vi "Data.vi"(7 "Data Type":T1(ring), 8 "Error In":errorcluster, 11 "Read Buffer":string) -> (0 "Error Out":errorcluster, 3 "XYZ":T2)   [LabVIEW 2010]
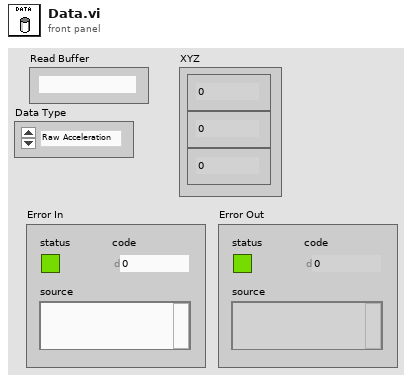
[diagram p1: front panel]
types:
  T1 = enum16{"Raw Acceleration", "Raw Gyro", "Complementy Filter", "Kalman Filter"}
  T2 = cluster{"Numeric Control":dbl, "Numeric Control":dbl, "Numeric Control":dbl}
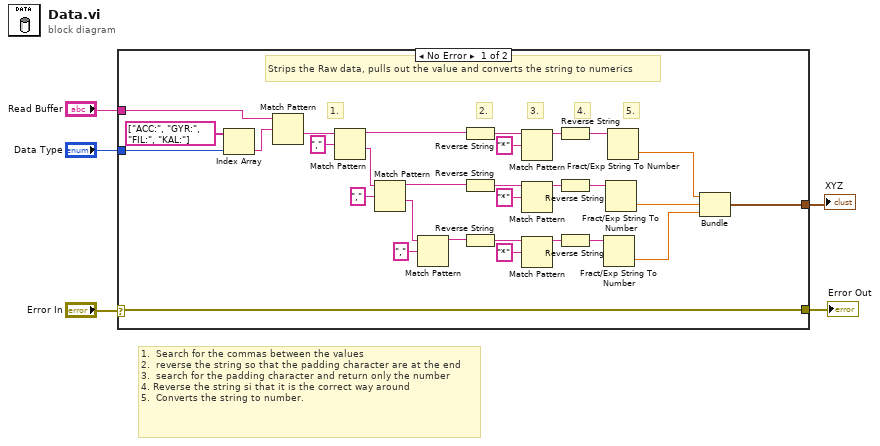
[diagram p0: block diagram]
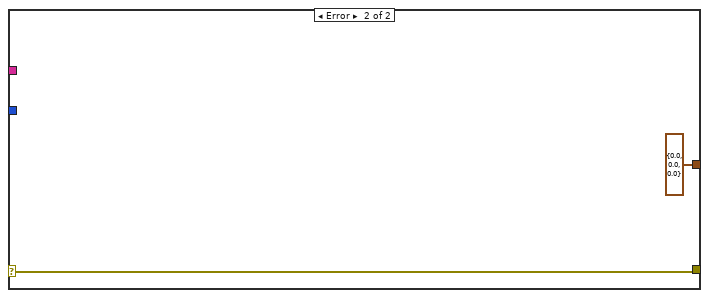
[diagram p2: hidden frame]
diagram:
  # "1.  Search for the commas between the values\n2.  reverse the string so that the padding character are at the end\n3.  search for the padding character and return only the number\n4. Reverse the string si that it is the correct way around\n5.  Converts the string to number."
  n1 = case shown="No Error" "Error In" {
    selector: "Error In" -> [w11 w37]
    tunnel: [w11 w37] -> w4
    tunnel: "Read Buffer" -> [w10 _]
    tunnel: [w9 cluster{dbl, dbl, dbl} {0.0, 0.0, 0.0}] -> w2
    tunnel: "Data Type" -> [w7 _]
    frame No Error {
      # "5."
      # "4."
      # "3."
      # "2."
      # "1."
      # "Strips the Raw data, pulls out the value and converts the string to numerics"
      n2 = Index Array(array=string[] ["ACC:", "GYR:", "FIL:", "KAL:"], index=w7) -> (element=w6:string)
      n3 = Match Pattern(string=w10, regular expression=w6) -> (after substring=w12:string)  [unwired: 1 in, 3 out]
      n4 = Match Pattern(string=w12, regular expression=",") -> (before substring=w14:string, after substring=w23:string)  [unwired: 1 in, 2 out]
      n5 = Match Pattern(string=w23, regular expression=",") -> (before substring=w21:string, after substring=w29:string)  [unwired: 1 in, 2 out]
      n6 = Match Pattern(string=w29, regular expression=",") -> (before substring=w25:string)  [unwired: 1 in, 3 out]
      n7 = Reverse String(1:w14) -> (0:w15:string)
      n8 = Reverse String(1:w21) -> (0:w20:string)
      n9 = Reverse String(1:w25) -> (0:w26:string)
      n10 = Match Pattern(string=w15, regular expression="*") -> (before substring=w17:string)  [unwired: 1 in, 3 out]
      n11 = Match Pattern(string=w20, regular expression="*") -> (before substring=w18:string)  [unwired: 1 in, 3 out]
      n12 = Match Pattern(string=w26, regular expression="*") -> (before substring=w28:string)  [unwired: 1 in, 3 out]
      n13 = Reverse String(1:w17) -> (0:w30:string)
      n14 = Reverse String(1:w18) -> (0:w31:string)
      n15 = Reverse String(1:w28) -> (0:w32:string)
      n16 = Fract/Exp String To Number(string=w32) -> (number=w35:dbl)  [unwired: 3 in, 1 out]
      n17 = Fract/Exp String To Number(string=w31) -> (number=w34:dbl)  [unwired: 3 in, 1 out]
      n18 = Fract/Exp String To Number(string=w30) -> (number=w33:dbl)  [unwired: 3 in, 1 out]
      n19 = Bundle(w33, w34, w35) -> (w9:cluster{dbl, dbl, dbl})  [unwired: 1 in]
    }
    frame Error {
    }
  }
  "Error Out" <- w4
  "XYZ" <- w2
